vi "Goal Position From Robot and Camera.vi"(0 "Targets":T1(array[cluster]), 1 "Pose X":dbl, 2 "Pose Y":dbl, 3 "Navx Yaw":dbl, 4 "servo angle":dbl) -> (5 "Goal X":dbl, 6 "Goal Y":dbl)   [LabVIEW 2016]
uses:
  <vilib>/Analysis/NI_AALBase.lvlib
  <vilib>/ptbypt/NI_PtbyPt.lvlib
panel:
  out "Average Y":dbl
  out "Height":dbl
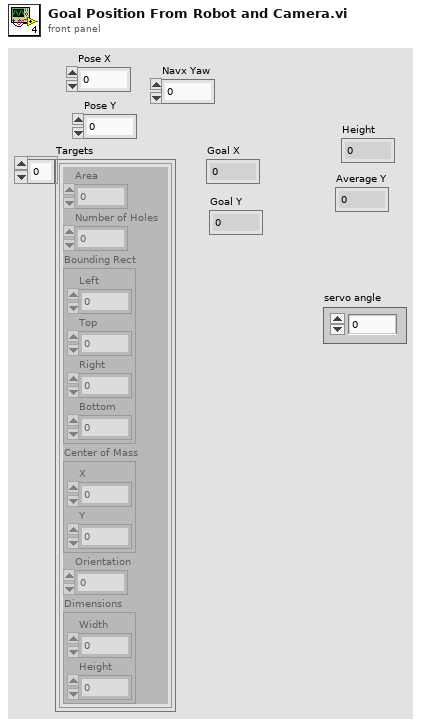
[diagram p1: front panel]
types:
  T1 = cluster{"Area":dbl, "Number of Holes":dbl, "Bounding Rect":cluster{"Left":dbl, "Top":dbl, "Right":dbl, "Bottom":dbl}, "Center of Mass":cluster{"X":dbl, "Y":dbl}, "Orientation":dbl, "Dimensions":cluster{"Width":dbl, "Height":dbl}}[]
  T2 = cluster{"Area":dbl, "Number of Holes":dbl, "Bounding Rect":cluster{"Left":dbl, "Top":dbl, "Right":dbl, "Bottom":dbl}, "Center of Mass":cluster{"X":dbl, "Y":dbl}, "Orientation":dbl, "Dimensions":cluster{"Width":dbl, "Height":dbl}}
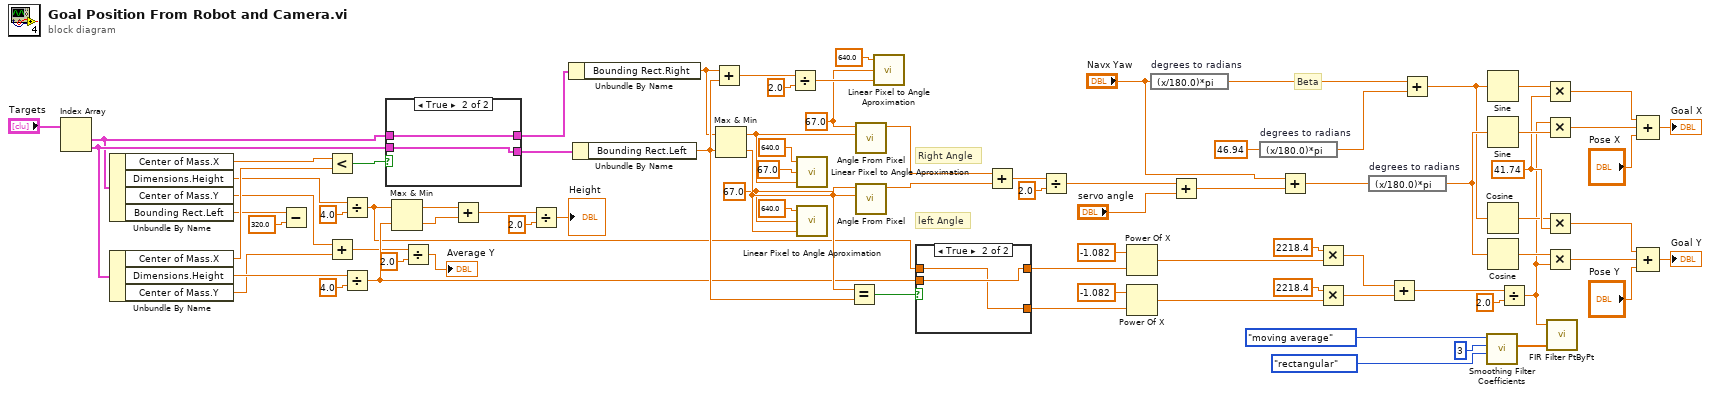
[diagram p0: block diagram]
diagram:
  w58 = 41.74 ("y")
  w64 = 67.0 ("Axis Fov")
  w63 = 67.0 ("Axis Fov")
  # "Beta"
  # "Right Angle"
  # "left Angle"
  n1 = Index Array(array="Targets") -> (element #1=w72:T2, element #2=w73:T2)  [unwired: 2 in]
  n2 = Unbundle By Name(w72) -> ("Center of Mass.X"=w70:dbl, "Dimensions.Height"=w34:dbl, "Center of Mass.Y"=w13:dbl, "Bounding Rect.Left"=w45:dbl)
  n3 = Unbundle By Name(w73) -> ("Center of Mass.X"=w77:dbl, "Dimensions.Height"=w36:dbl, "Center of Mass.Y"=w12:dbl)
  n4 = Subtract(x=w45, y=320.0) -> ()  [unwired: 1 out]
  n5 = Less?(x=w70, y=w77) -> (x < y?=w71:bool)
  n6 = Add(x=w13, y=w12) -> (x+y=w15:dbl)
  n7 = Divide(x=w34, y=4.0) -> (x/y=w33:dbl)
  n8 = Divide(x=w36, y=4.0) -> (x/y=w37:dbl)
  n9 = case shown="True" w71 {
    tunnel: w72 -> [w85 w88]
    tunnel: [w86 w88] -> w74
    tunnel: w73 -> [w86 w87]
    tunnel: [w85 w87] -> w75
    frame False {
    }
    frame True {
    }
  }
  n10 = Max & Min(x=w33, y=w37) -> (max(x,y)=w20:dbl, min(x,y)=w19:dbl)
  n11 = Divide(x=w15, y=2.0) -> (x/y=→"Average Y":dbl)
  n12 = Add(x=w20, y=w19) -> (x+y=w21:dbl)
  n13 = Divide(x=w21, y=2.0) -> (x/y=→"Height":dbl)
  n14 = Unbundle By Name(w74) -> ("Bounding Rect.Right"=w76:dbl)
  n15 = Unbundle By Name(w75) -> ("Bounding Rect.Left"=w78:dbl)
  n16 = Add(x=w76, y=w78) -> (x+y=w23:dbl)
  n17 = Max & Min(x=w76, y=w78) -> (max(x,y)=w68:dbl, min(x,y)=w65:dbl)
  n18 = Divide(x=w23, y=2.0) -> (x/y=w67:dbl)
  n19 = call "Linear Pixel to Angle Aproximation.vi"("Axis Pixel"=w68, "Axis Fov"=67.0, "Axis Lengh"=640.0) -> ()  [unwired: 1 out]
  n20 = call "Linear Pixel to Angle Aproximation.vi"("Axis Pixel"=w65, "Axis Fov"=w64, "Axis Lengh"=640.0) -> ()  [unwired: 1 out]
  n21 = Equal?(x=w65, y=w78) -> (x = y?=w28:bool)
  n22 = call "Angle From Pixel.vi"("Pixel"=w68, "Angle Aperture"=w63) -> ("Theta"=w69:dbl)  [unwired: 9 in]
  n23 = call "Angle From Pixel.vi"("Pixel"=w65, "Angle Aperture"=w64) -> ("Theta"=w66:dbl)  [unwired: 9 in]
  n24 = call "Linear Pixel to Angle Aproximation.vi"("Axis Pixel"=w67, "Axis Fov"=w63, "Axis Lengh"=640.0) -> ()  [unwired: 1 out]
  n25 = case shown="True" w28 {
    tunnel: w37 -> [w89 w92]
    tunnel: [w90 w92] -> w43
    tunnel: w33 -> [w90 w91]
    tunnel: [w89 w91] -> w39
    frame False {
    }
    frame True {
    }
  }
  n26 = Add(x=w69, y=w66) -> (x+y=w50:dbl)
  n27 = Divide(x=w50, y=2.0) -> (x/y=w3:dbl)
  n28 = Power Of X(1:w43, 2:-1.082 ("x")) -> (0:w42:dbl)
  n29 = Power Of X(1:w39, 2:-1.082 ("x")) -> (0:w25:dbl)
  n30 = expression code="(x/180.0)*pi" "degrees to radians"("Navx Yaw") -> (w17:dbl)
  n31 = Add(x=w3, y="servo angle") -> (x+y=w2:dbl)
  n32 = expression code="(x/180.0)*pi" "degrees to radians"(46.94 ("Axis Lengh")) -> (w5:dbl)
  n33 = Add(x="Navx Yaw", y=w2) -> (x+y=w61:dbl)
  n34 = Multiply(x=2218.4, y=w42) -> (x*y=w46:dbl)
  n35 = Multiply(x=2218.4, y=w25) -> (x*y=w51:dbl)
  n36 = expression code="(x/180.0)*pi" "degrees to radians"(w61) -> (w62:dbl)
  n37 = Add(x=w46, y=w51) -> (x+y=w47:dbl)
  n38 = Add(x=w17, y=w5) -> (x+y=w16:dbl)
  n39 = call <vilib>:"Smoothing Filter Coefficients.vi"("shape"=enum16{"rectangular", "triangular"}."rectangular", "half-width"=3, "type"=enum16{"moving average", "exponential"}."moving average") -> ("forward coefficients"=w10:dbl[])  [unwired: 6 in, 2 out]
  n40 = Sine(x=w16) -> (sin(x)=w57:dbl)
  n41 = Sine(x=w62) -> (sin(x)=w59:dbl)
  n42 = Cosine(x=w16) -> (cos(x)=w52:dbl)
  n43 = Cosine(x=w62) -> (cos(x)=w55:dbl)
  n44 = Divide(x=w47, y=2.0) -> (x/y=w4:dbl)
  n45 = Multiply(x=w57, y=w58) -> (x*y=w56:dbl)
  n46 = Multiply(x=w4, y=w59) -> (x*y=w60:dbl)
  n47 = Multiply(x=w52, y=w58) -> (x*y=w53:dbl)
  n48 = Multiply(x=w55, y=w4) -> (x*y=w54:dbl)
  n49 = call <vilib>:"FIR Filter PtByPt.vi"("Forward Coefficients"=w10, "x"=w4) -> ()  [unwired: 2 in, 2 out]
  n50 = Compound Arithmetic op=ADD(w56, w60, "Pose X") -> (→"Goal X":dbl)
  n51 = Compound Arithmetic op=ADD(w53, w54, "Pose Y") -> (→"Goal Y":dbl)
